vi "AttCtrlThruster.vi"(0 "ctclk":bool, 1 "Duty Cycle":dbl=1.0, 2 "Up":bool, 3 "Period":dbl=25.0, 4 "clkwis":bool, 5 "Float":bool, 6 "Angular Acceleration":u16(ring) items=["Fast", "Slow"], 7 "Left":bool, 8 "Right":bool, 9 "task in":refnum<k21>, 11 "error in":errorcluster, 13 "Down":bool) -> (10 "task out":refnum<k21>, 15 "error out":errorcluster)   [LabVIEW 2012]
panel:
  # "Attitude Control"
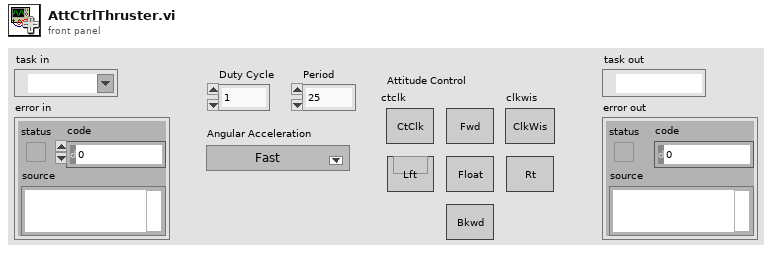
[diagram p1: front panel]
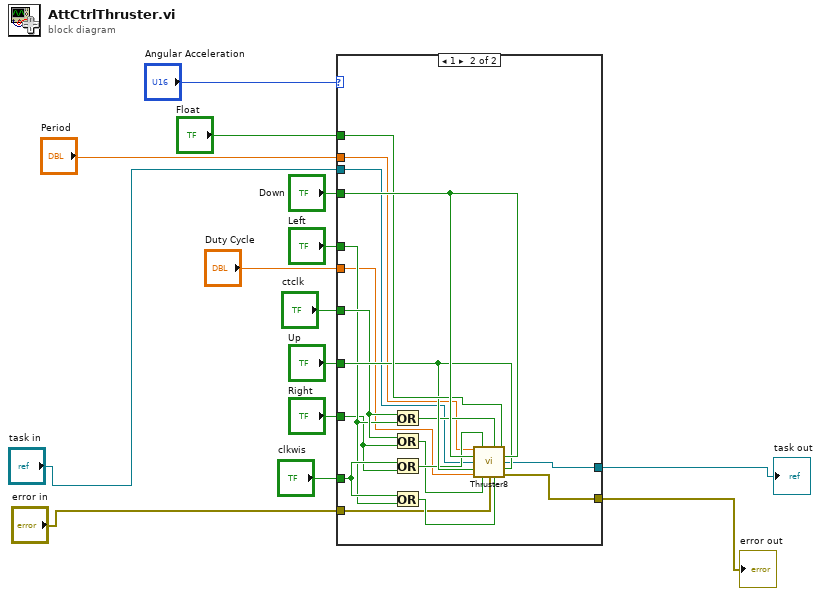
[diagram p0: block diagram]
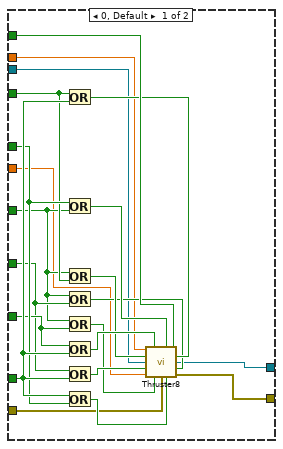
[diagram p2: hidden frame]
diagram:
  n1 = case shown="1" "Angular Acceleration" {
    tunnel: "Float" -> [w35 w51]
    tunnel: "Down" -> [w27 w52]
    tunnel: "Left" -> [w29 w45]
    tunnel: "Up" -> [w23 w50]
    tunnel: "Right" -> [w25 w43]
    tunnel: "clkwis" -> [w31 w49]
    tunnel: "ctclk" -> [w22 w46]
    tunnel: "Duty Cycle" -> [w20 w41]
    tunnel: "Period" -> [w19 w40]
    tunnel: "task in" -> [w18 w38]
    tunnel: "error in" -> [w17 w39]
    tunnel: [w16 w37] -> w4
    tunnel: [w15 w36] -> w3
    frame 0, Default {
      n2 = Or(x=w27, y=w31) -> (x .or. y?=w30:bool)
      n3 = Or(x=w29, y=w22) -> (x .or. y?=w28:bool)
      n4 = Or(x=w22, y=w27) -> (x .or. y?=w26:bool)
      n5 = Or(x=w22, y=w23) -> (x .or. y?=w21:bool)
      n6 = Or(x=w22, y=w25) -> (x .or. y?=w24:bool)
      n7 = Or(x=w25, y=w31) -> (x .or. y?=w33:bool)
      n8 = Or(x=w23, y=w31) -> (x .or. y?=w34:bool)
      n9 = Or(x=w31, y=w29) -> (x .or. y?=w32:bool)
      n10 = call "Thruster8.vi"("period"=w19, "Thruster 2"=w33, "Truster1"=w28, "Floating"=w35, "Thruster 3"=w26, "Thruster 8"=w30, "task in"=w18, "Thruster 4"=w34, "Thruster 7"=w21, "Duty Cycle"=w20, "Thruster 5"=w24, "error in"=w17, "Thruster 6"=w32) -> ("task out"=w16:refnum<k21>, "error out"=w15:errorcluster)  [unwired: 1 in]
    }
    frame 1 {
      n11 = Or(x=w46, y=w45) -> (x .or. y?=w44:bool)
      n12 = Or(x=w46, y=w43) -> (x .or. y?=w42:bool)
      n13 = Or(x=w49, y=w43) -> (x .or. y?=w48:bool)
      n14 = Or(x=w49, y=w45) -> (x .or. y?=w47:bool)
      n15 = call "Thruster8.vi"("period"=w40, "Thruster 2"=w48, "Truster1"=w44, "Floating"=w51, "Thruster 3"=w52, "Thruster 8"=w52, "task in"=w38, "Thruster 4"=w50, "Thruster 7"=w50, "Duty Cycle"=w41, "Thruster 5"=w42, "error in"=w39, "Thruster 6"=w47) -> ("task out"=w37:refnum<k21>, "error out"=w36:errorcluster)  [unwired: 1 in]
    }
  }
  "task out" <- w4
  "error out" <- w3
